vi "SVN ok.vi"(10 "error in":errorcluster, 11 "SVN in":T1) -> (2 "error out":errorcluster, 3 "SVN ok":bool)   [LabVIEW 2012]
uses:
  SVN.ctl
  Which method type.ctl
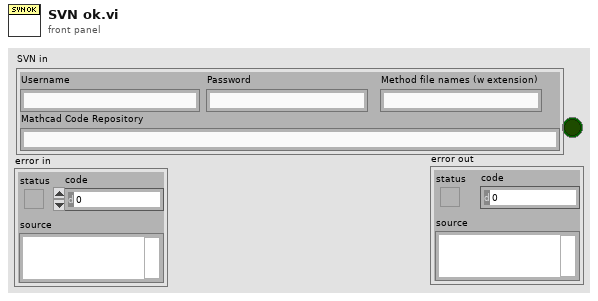
[diagram p1: front panel]
types:
  T1 = typedef "SVN.ctl" = cluster{"Mathcad Code Repository":string, "Username":string, "Password":string, "Method file names (w extension)":string}
  T2 = typedef "Which method type.ctl" = enum16{"Master Method", "Method"}
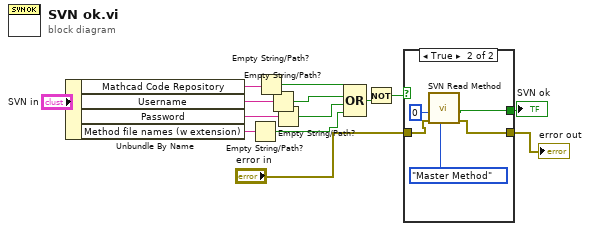
[diagram p0: block diagram]
diagram:
  n1 = Unbundle By Name("SVN in") -> ("Mathcad Code Repository"=w14:string, "Username"=w13:string, "Password"=w12:string, "Method file names (w extension)"=w2:string)
  n2 = Empty String/Path?(string/path=w2) -> (empty?=w1:bool)
  n3 = Empty String/Path?(string/path=w14) -> (empty?=w11:bool)
  n4 = Empty String/Path?(string/path=w13) -> (empty?=w10:bool)
  n5 = Empty String/Path?(string/path=w12) -> (empty?=w9:bool)
  n6 = Compound Arithmetic op=OR(w11, w10, w9, w1) -> (w8:bool)
  n7 = Not(x=w8) -> (.not. x?=w7:bool)
  n8 = case shown="True" w7 {
    selector: w7 -> [w16 _]
    tunnel: "error in" -> [w15 w21]
    tunnel: [w16 w20] -> w6
    tunnel: [w15 w19] -> w3
    frame False {
    }
    frame True {
      n9 = call "SVN Read Method.vi"("Which Method Type"=Which_method_type."Master Method", "error in (no error)"=w21, "Method version"=0) -> ("error out"=w19:errorcluster, "Valid method"=w20:bool)  [unwired: 6 in, 1 out]
    }
  }
  "SVN ok" <- w6
  "error out" <- w3
